vi "Plot.vi"(2 "Zen Analytics in":refnum<class "Zen Analytics.lvclass">, 3 "IndexOfMeasurement":i32, 6 "InitializationValue-Input-Barplot":T1, 7 "InitializationValue-Input-PieCahrt":T1, 8 "error Input":errorcluster, 9 "Initialization input":dbl[][](array[numeric]), 10 "Graph Refference's":T3, 11 "Plot Cluster":T2) -> (0 "error output":errorcluster, 1 "InitializationOutput":dbl[][](array[numeric]), 4 "InitializationValue-output-Barplot":T1, 5 "InitializationValue-output-PieCahrt":T1)   [LabVIEW 2019, in "Zen Analytics.lvlib" / "Zen Analytics.lvclass"]
uses:
  Zen Analytics.lvclass
  Dependency/GraphReff.ctl
  Dependency/Plot Cluster.ctl
panel:
  # "s"
  # "ANALYTICS DASHBOARD"
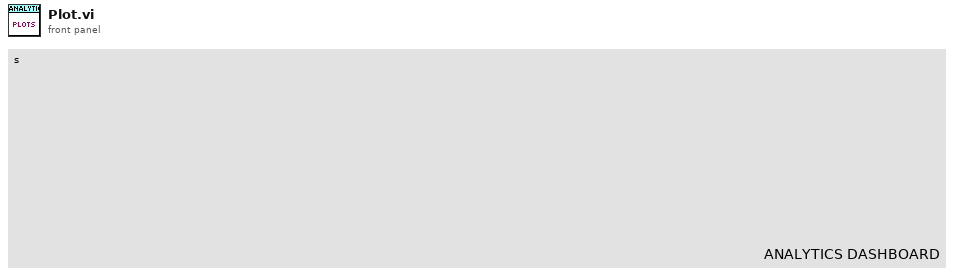
[diagram p1: front panel]
types:
  T1 = cluster{"InitializationDefect":dbl[], "InitializationProduction":dbl[]}
  T2 = typedef "Zen Analytics.lvlib/Zen Analytics.lvclass/Plot Cluster.ctl" = cluster{"Reduced 2D":dbl[][], "Start Index":i32, "No Of New Termnals":i32, "Top/Bottom":bool, "Values Inserted":i32, "Re-Initialised":bool, "Statistical params":string[][], "MeasurementInitializationData":cluster{"Measurement-ID":i32[], "Measurement Names":string[], "NominalValues":dbl[], "LSL":dbl[], "USL":dbl[], "LCL":dbl[], "UCL":dbl[]}, "MeasurementData":cluster{"Measurement ID":i32, "Measurement Name":string, "Nominal Values":dbl, "LSL":dbl, "USL":dbl, "LCL":dbl, "UCL":dbl}[], "ResultData2D":dbl[][], "PlotParameters":cluster{"Trend":cluster{"TrendPlotID":dbl, "PlotProperties":cluster{"FontName":string, "FontSize":dbl, "FontColor":string, "IsBold":bool, "IsItalic":bool, "PlotColor":string}}[], "Histogram":cluster{"HistogramPlotID":dbl, "PlotProperties":cluster{"FontName":string, "FontSize":dbl, "FontColor":string, "IsBold":bool, "IsItalic":bool, "PlotColor":string}}[], "BarPlot":cluster{"BarPlotID":dbl, "BarValuesID":dbl, "PlotProperties":cluster{"FontName":string, "FontSize":dbl, "IsBold":bool, "IsItalic":bool, "FontColor":string}, "Sectors":string[]}[], "PieChart":cluster{"PieChartID":dbl, "PieChartValueID":dbl, "PlotProperties":cluster{"FontName":string, "FontSize":dbl, "IsBold":bool, "IsItalic":bool, "FontColor":string}, "Sectors":string[]}[]}}
  T3 = typedef "Zen Analytics.lvlib/Zen Analytics.lvclass/GraphReff.ctl" = cluster{"HistgramGraph-reff":refnum<vi>[], "BarGraph-reff":refnum<vi>[], "PieGraph-reff":refnum<vi>[], "Lable-reff":refnum<vi>[], "TrendGraph-reff":refnum<vi>[], "CpCpkTable":refnum<vi>}
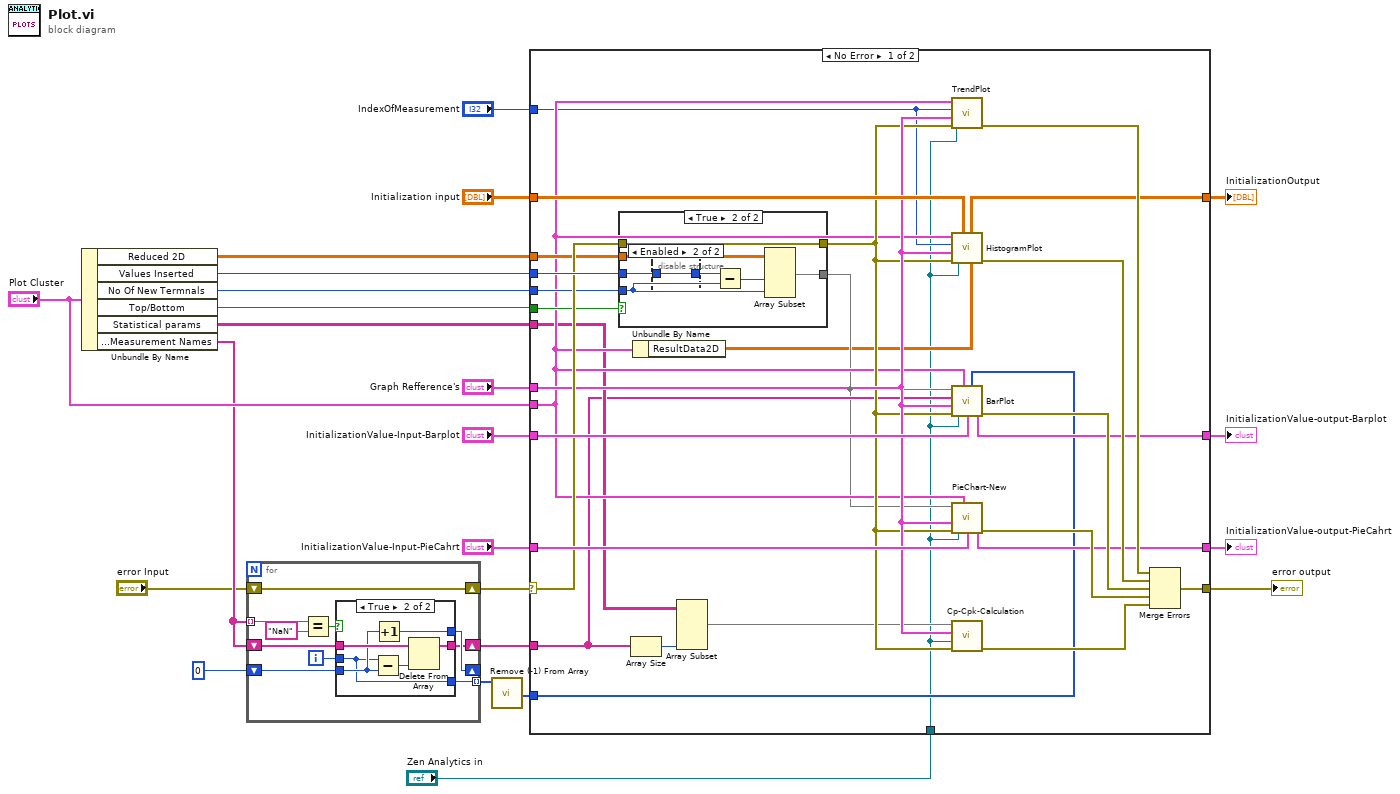
[diagram p0: block diagram]
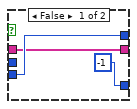
[diagram p2: hidden frame]
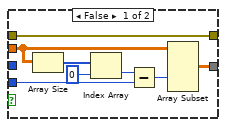
[diagram p3: hidden frame]
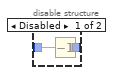
[diagram p4: hidden frame]
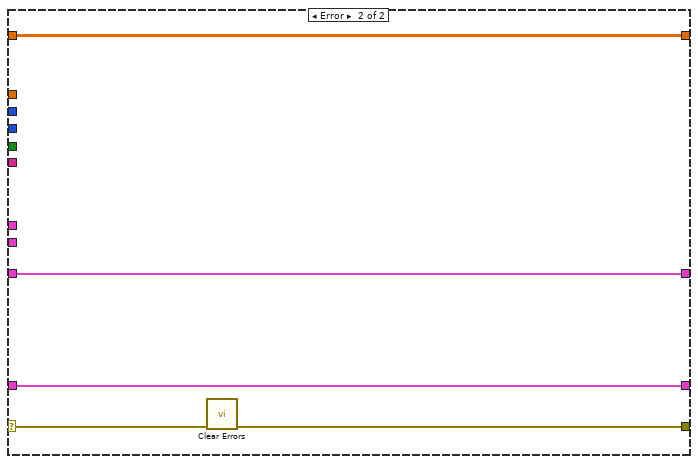
[diagram p5: hidden frame]
diagram:
  n1 = Unbundle By Name("Plot Cluster") -> ("Reduced 2D"=w23:dbl[][], "Values Inserted"=w17:i32, "No Of New Termnals"=w15:i32, "Top/Bottom"=w16:bool, "Statistical params"=w11:string[][], "MeasurementInitializationData.Measurement Names"=w9:string[])
  n2 = for {
    tunnel: w9 -> [w27] mode=indexing
    shift-right: [w32] -> _
    shift-left: 0 -> [w33]
    shift-right: [w29] -> w7
    shift-left: w9 -> [w30]
    tunnel: [w25] -> w6 mode=indexing
    shift-right: [w24] -> w4
    shift-left: "error Input" -> [w24]
    i -> [w31]
    n3 = Equal?(x=w27, y="NaN") -> (x = y?=w26:bool)
    n4 = case shown="True" w26 {
      tunnel: w30 -> [w35 w42]
      tunnel: w33 -> [w36 w38]
      tunnel: [w36 w40] -> w32
      tunnel: [w35 w41] -> w29
      tunnel: w31 -> [_ w37]
      tunnel: [-1 w37] -> w25
      frame False {
      }
      frame True {
        n5 = Subtract(x=w37, y=w38) -> (x-y=w39:i32)
        n6 = Increment(x=w38) -> (x+1=w40:i32)
        n7 = Delete From Array(array=w42, index=w39) -> (array with subset deleted=w41:string[])  [unwired: 1 in, 1 out]
      }
    }
  }
  n8 = call "Remove (-1) From Array.vi"("Input"=w6) -> ("Output"=w5:i32[])  [unwired: 10 in]
  n9 = case shown="No Error" w4 {
    selector: w4 -> [w61 w94]
    tunnel: [w68 w90] -> w2
    tunnel: w23 -> [w56 _]
    tunnel: "Graph Refference's" -> [w57 _]
    tunnel: [w66 w93] -> w19
    tunnel: "InitializationValue-Input-Barplot" -> [w65 w93]
    tunnel: "InitializationValue-Input-PieCahrt" -> [w64 w92]
    tunnel: [w63 w92] -> w18
    tunnel: w16 -> [w54 _]
    tunnel: w15 -> [w53 _]
    tunnel: w17 -> [w62 _]
    tunnel: "Plot Cluster" -> [w52 _]
    tunnel: "Initialization input" -> [w60 w91]
    tunnel: [w59 w91] -> w12
    tunnel: w11 -> [w51 _]
    tunnel: w7 -> [w48 _]
    tunnel: "IndexOfMeasurement" -> [w47 _]
    tunnel: w5 -> [w46 _]
    tunnel: "Zen Analytics in" -> [w43 _]
    frame No Error {
      n10 = case shown="True" w54 {
        tunnel: w56 -> [w75 w86]
        tunnel: [w74 w85] -> w45
        tunnel: w53 -> [w73 w83]
        tunnel: w62 -> [_ w82]
        tunnel: w61 -> [w72 w80]
        tunnel: [w72 w80] -> w55
        frame False {
          n11 = Array Size(array=w75) -> (size(s)=w79:i32[])
          n12 = Index Array(array=w79, index=0) -> (element=w77:i32)
          n13 = Subtract(x=w77, y=w73) -> (x-y=w76:i32)
          n14 = Array Subset(array=w75, index (row)=w76) -> (w74:dbl[][])  [unwired: 3 in]
        }
        frame True {
          n15 = disable-structure shown="Enabled" {
            disable-tunnel: w82 -> [w88 w89]
            disable-tunnel: [w87 w89] -> w81
            frame Disabled {
              n16 = Decrement(x=w88) -> (x-1=w87:i32)
            }
            frame Enabled {
            }
          }
          n17 = Subtract(x=w81, y=w83) -> (x-y=w84:i32)
          n18 = Array Subset(array=w86, index (row)=w84, length (row)=w83) -> (w85:dbl[][])  [unwired: 2 in]
        }
      }
      n19 = Array Size(array=w48) -> (size(s)=w49:i32)
      n20 = Unbundle By Name(w52) -> ("ResultData2D"=w44:dbl[][])
      n21 = Array Subset(array=w51, length (col)=w49) -> (w50:string[][])  [unwired: 3 in]
      n22 = call "TrendPlot.vi"("Zen Analytics in"=w43, "error in (no error)"=w55, "Graph Refference's"=w57, "IndexOfMeasurement"=w47, "Plot Cluster"=w52) -> ("error out"=w67:errorcluster)  [unwired: 6 in]
      n23 = call "HistogramPlot.vi"("Zen Analytics in"=w43, "Reduced 2D"=w44, "Initialization input"=w60, "error in (no error)"=w55, "Graph Refference's"=w57, "IndexOfMeasurement"=w47, "Plot Cluster"=w52) -> ("error out"=w71:errorcluster, "InitializationOutput"=w59:dbl[][])  [unwired: 3 in]
      n24 = call "BarPlot.vi"("Zen Analytics in"=w43, "MeasuremetDisabledIndex"=w46, "InitializationValue-Input"=w65, "Plot Cluster"=w52, "error in (no error)"=w55, "Graph Refference's"=w57, "MeasurementInitializationData.Measurement Names"=w48, "Input_Data"=w45) -> ("error out"=w70:errorcluster, "InitializationValues-Output"=w66:T1)  [unwired: 2 in]
      n25 = call "PieChart-New.vi"("InitializationValue-Input"=w64, "Plot Cluster"=w52, "error in (no error)"=w55, "Graph Refference's"=w57, "Zen Analytics in"=w43, "Input_Data"=w45) -> ("error out"=w69:errorcluster, "InitializationValues-Output"=w63:T1)  [unwired: 4 in]
      n26 = call "Cp-Cpk-Calculation.vi"("Zen Analytics in"=w43, "error in (no error)"=w55, "Graph Refference's"=w57, "Statistical params"=w50) -> ("error out"=w58:errorcluster)  [unwired: 7 in]
      n27 = Merge Errors(w67, w71, w70, w69, w58) -> (w68:errorcluster)
    }
    frame Error {
      n28 = call <vilib>:"Clear Errors.vi"("error in (no error)"=w94) -> ("error out"=w90:errorcluster)  [unwired: 5 in, 1 out]
    }
  }
  "error output" <- w2
  "InitializationValue-output-Barplot" <- w19
  "InitializationValue-output-PieCahrt" <- w18
  "InitializationOutput" <- w12
